vi "MeasureMessage.vi"() -> ()   [LabVIEW 2017]
uses:
  MeasureMessage.ctl
panel:
  in  "MeasureMessage":T1
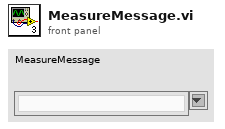
[diagram p1: front panel]
types:
  T1 = typedef "MeasureMessage.ctl" = string
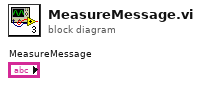
[diagram p0: block diagram]
diagram:
